vi "Update Caller.vi"(8 "error in (no error)":errorcluster, 9 "New Values":cluster{"Fan A":T1, "Fan B":T1}, 10 "Old Values":cluster{"Fan A":T1, "Fan B":T1}, 11 "Dual Fan":refnum<class "Dual Fan.lvclass">) -> (0 "error out":errorcluster)   [LabVIEW 2025, in "Dual Fan.lvlib" / "Dual Fan.lvclass"]
uses:
  Dual Fan.lvclass
  C:/Program Files/National Instruments/LabVIEW 2025/vi.lib/ActorFramework/Actor/Actor.lvclass
  Fan Info.ctl
  <vilib>/ActorFramework/Actor/Actor.lvclass/Actor.ctl
  Dual Fan.lvclass/Dual Fan.ctl
  Update Fan Status Msg/Update Fan Status Msg.lvclass/Update Fan Status Msg.ctl
  <vilib>/ActorFramework/Message Enqueuer/Message Enqueuer.lvclass/Message Enqueuer.ctl
  <vilib>/ActorFramework/Message Enqueuer/Enqueue.vi
  Update Fan Status Msg/Update Fan Status Msg.lvclass
  C:/Program Files/National Instruments/LabVIEW 2025/vi.lib/ActorFramework/Message/Message.lvclass
  <vilib>/ActorFramework/Message Priority Queue/Priority Enqueue.vi
  <vilib>/ActorFramework/Actor/Actor.lvclass
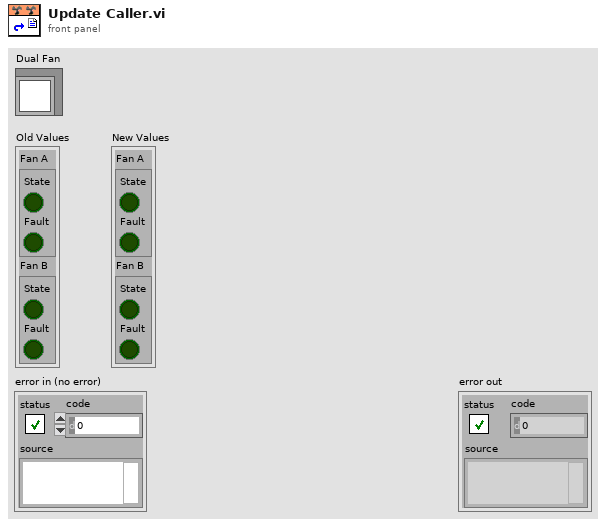
[diagram p1: front panel]
types:
  T1 = typedef "Dual Fan.lvlib/Dual Fan.lvclass/Fan Info.ctl" = cluster{"State":bool, "Fault":bool}
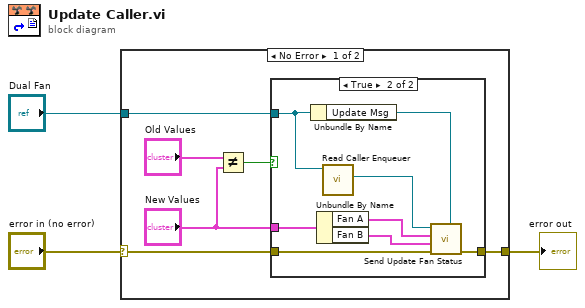
[diagram p0: block diagram]
diagram:
  n1 = case shown="No Error" "error in (no error)" {
    selector: "error in (no error)" -> [w8 w19]
    tunnel: [w7 w19] -> w2
    tunnel: "Dual Fan" -> [w9 _]
    frame No Error {
      n2 = Not Equal?(x="Old Values", y="New Values") -> (x != y?=w5:bool)
      n3 = case shown="True" w5 {
        tunnel: w9 -> [_ w18]
        tunnel: w8 -> [w10 w15]
        tunnel: [w10 w14] -> w7
        tunnel: "New Values" -> [_ w13]
        frame False {
        }
        frame True {
          n4 = Unbundle By Name(w18) -> ("Update Msg"=w16:refnum<class "Update Fan Status Msg.lvclass">)
          n5 = Unbundle By Name(w13) -> ("Fan A"=w12:T1, "Fan B"=w11:T1)
          n6 = call <vilib>:"Read Caller Enqueuer.vi"("Actor"=w18) -> ("Caller Enqueuer"=w17:refnum<class "Message Enqueuer.lvclass">)  [unwired: 10 in]
          n7 = call "Send Update Fan Status.vi"("Update Msg Object"=w16, "error in (no error)"=w15, "Fan B"=w11, "Fan A"=w12, "Message Enqueuer"=w17) -> ("error out"=w14:errorcluster)  [unwired: 6 in]
        }
      }
    }
    frame Error {
    }
  }
  "error out" <- w2
